vi "Measurement UI.vi"() -> ()   [LabVIEW 2023, in "FPT Framework UI.lvlib"]
uses:
  FPT Framework UI.lvlib
panel:
  in  "Measurement Graph":T1(tab)
  out "General Graph 1":T2(graph)
  out "General Graph 2":T2(graph)
  out "General Graph 3":T2(graph)
  out "General Graph 4":T2(graph)
  out "General Graph 5":T2(graph)
  out "PAE@Pin(s)":string[](array[string])
  out "Gain@Pin(s)":string[](array[string])
  out "Pout@Pin(s)":string[](array[string])
  out "Pout@Pin vs Freq":dbl[][](array[numeric])
  out "PAE vs Pin per Freq":dbl[][](array[numeric])
  out "Gain vs Pin per Freq":dbl[][](array[numeric])
  out "Group B Graph":refnum<vi>[](array[refnum])
  out "Group A Graph":refnum<vi>[](array[refnum])
  in  "Power sequencing file path":string
  out "All Graph Refs":refnum<vi>[](array[refnum])
  out "Pout vs Pin per Freq":dbl[][](array[numeric])
  out "OPxdB vs Freq":dbl[][](array[numeric])
  out "Linear Gain vs Freq":dbl[][](array[numeric])
  out "Frequencies":string[](array[string])
  out "OPxdB(s)":string[](array[string])
  out "Linear Gain(s)":string[](array[string])
  out "Full Data per Frequency":string[][](array[string])
  out "Pin(s)":string[](array[string])
  in  "SMU name":string caption="SMU Name"
  out "Table 2 Header":string[](array[string])
  out "Table 1 Header":string[](array[string])
  out "Gain@Pin vs Freq":dbl[][](array[numeric])
  out "PAE@Pin vs Freq":dbl[][](array[numeric])
  out "MeasTable 1":string[][](table)
  out "MeasTable 2":string[][](table)
  in  "Mode of operation":enum32{"Power Sequence", "Measurement 1"}(ring) caption="Configuration"
  in  "Tab Control":enum32{"Power Sequence", "Measurement 1"}(tab)
  in  "Power sequencing file path_update":path caption="Power Sequencing File Path"
  in  "SMU channel":string caption="SMU Channel"
  in  "SMU name_update":refnum<k15> caption="SMU Name"
  in  "Compression_Target Pin (dBm)":dbl=1.0 caption="Target Pin" format="%#pdBm"
  in  "Compression_Expected DUT Gain (dB)":dbl=17.5 caption="Expected DUT Gain" format="%#pdB"
  in  "Compression_Max Linear Range (dBm)":dbl=-10.0 caption="Max Linear Range" format="%#pdBm"
  in  "Compression_Compression Point (dB)":dbl=1.0 caption="PxdB" format="%#pdB"
  in  "Compression_RFSG Frequency Start (Hz)":dbl=6000000000.0 caption="Frequency Start" step=1000000.0 format="%#pHz"
  in  "Compression_RFSG Power Start (dBm)":dbl=-20.0 caption="Power Start" format="%#pdBm"
  in  "Compression_RFSG Power Step Size (dB)":dbl=1.0 caption="Power Step Size" format="%#pdB"
  in  "Compression_RFSG Power Stop(dBm)":dbl=4.0 caption="Power End" format="%#pdBm"
  in  "Compression_RBW (Hz)":dbl=5000000.0 caption="RBW" format="%#pHz"
  in  "Compression_RFSG Frequency Stop (Hz)":dbl=18000000000.0 caption="Frequency Stop" step=1000000.0 format="%#pHz"
  in  "Compression_RFSG Number of Frequency Step":i32=10 caption="Number of Steps"
  out "Status":string
  # "Frequency Sweep"
  # "Power Sweep"
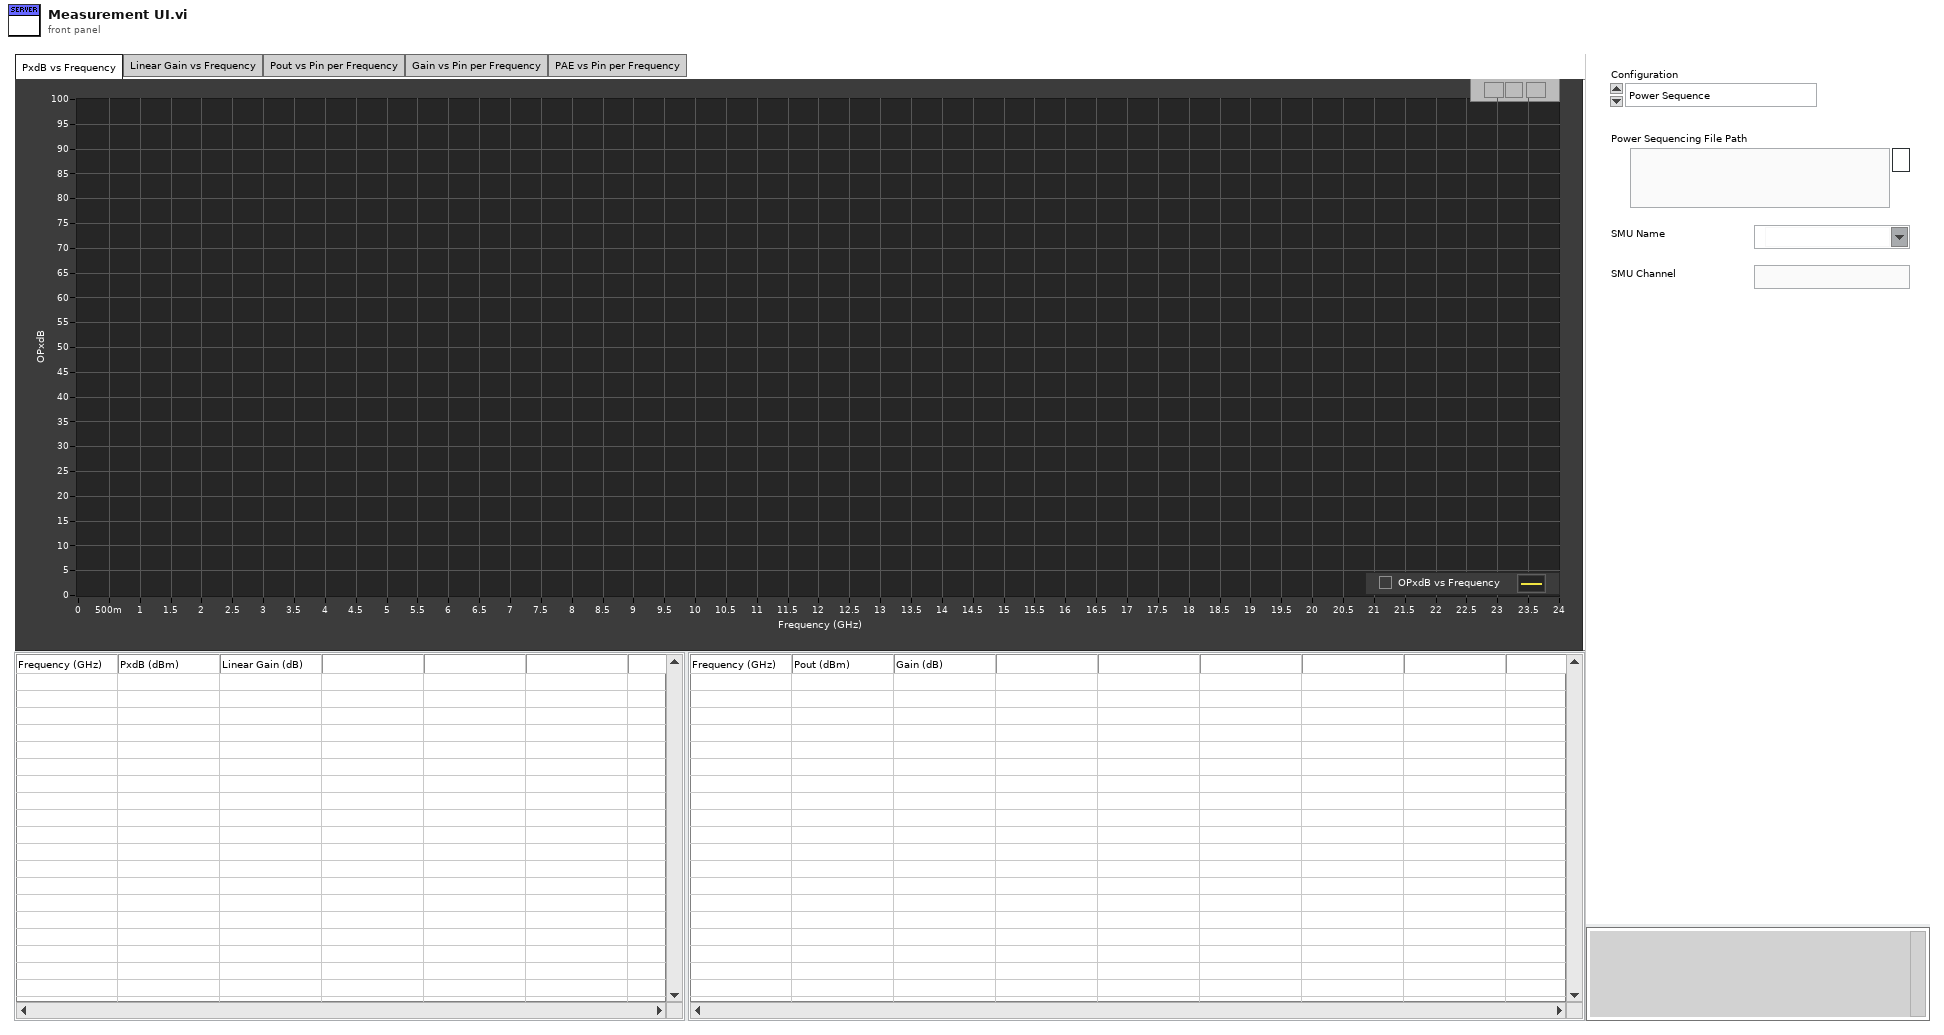
[diagram p1: front panel]
types:
  T1 = enum32{"PxdB vs Frequency", "Linear Gain vs Frequency", "Pout vs Pin per Frequency", "Gain vs Pin per Frequency", "PAE vs Pin per Frequency", "Hidden Controls"}
  T2 = cluster{"Load currents":dbl[], "Efficiency":dbl[]}[]
  T3 = cluster{"Shift":bool, "Ctrl":bool, "Alt":bool, "Cmd":bool, "Opt":bool}
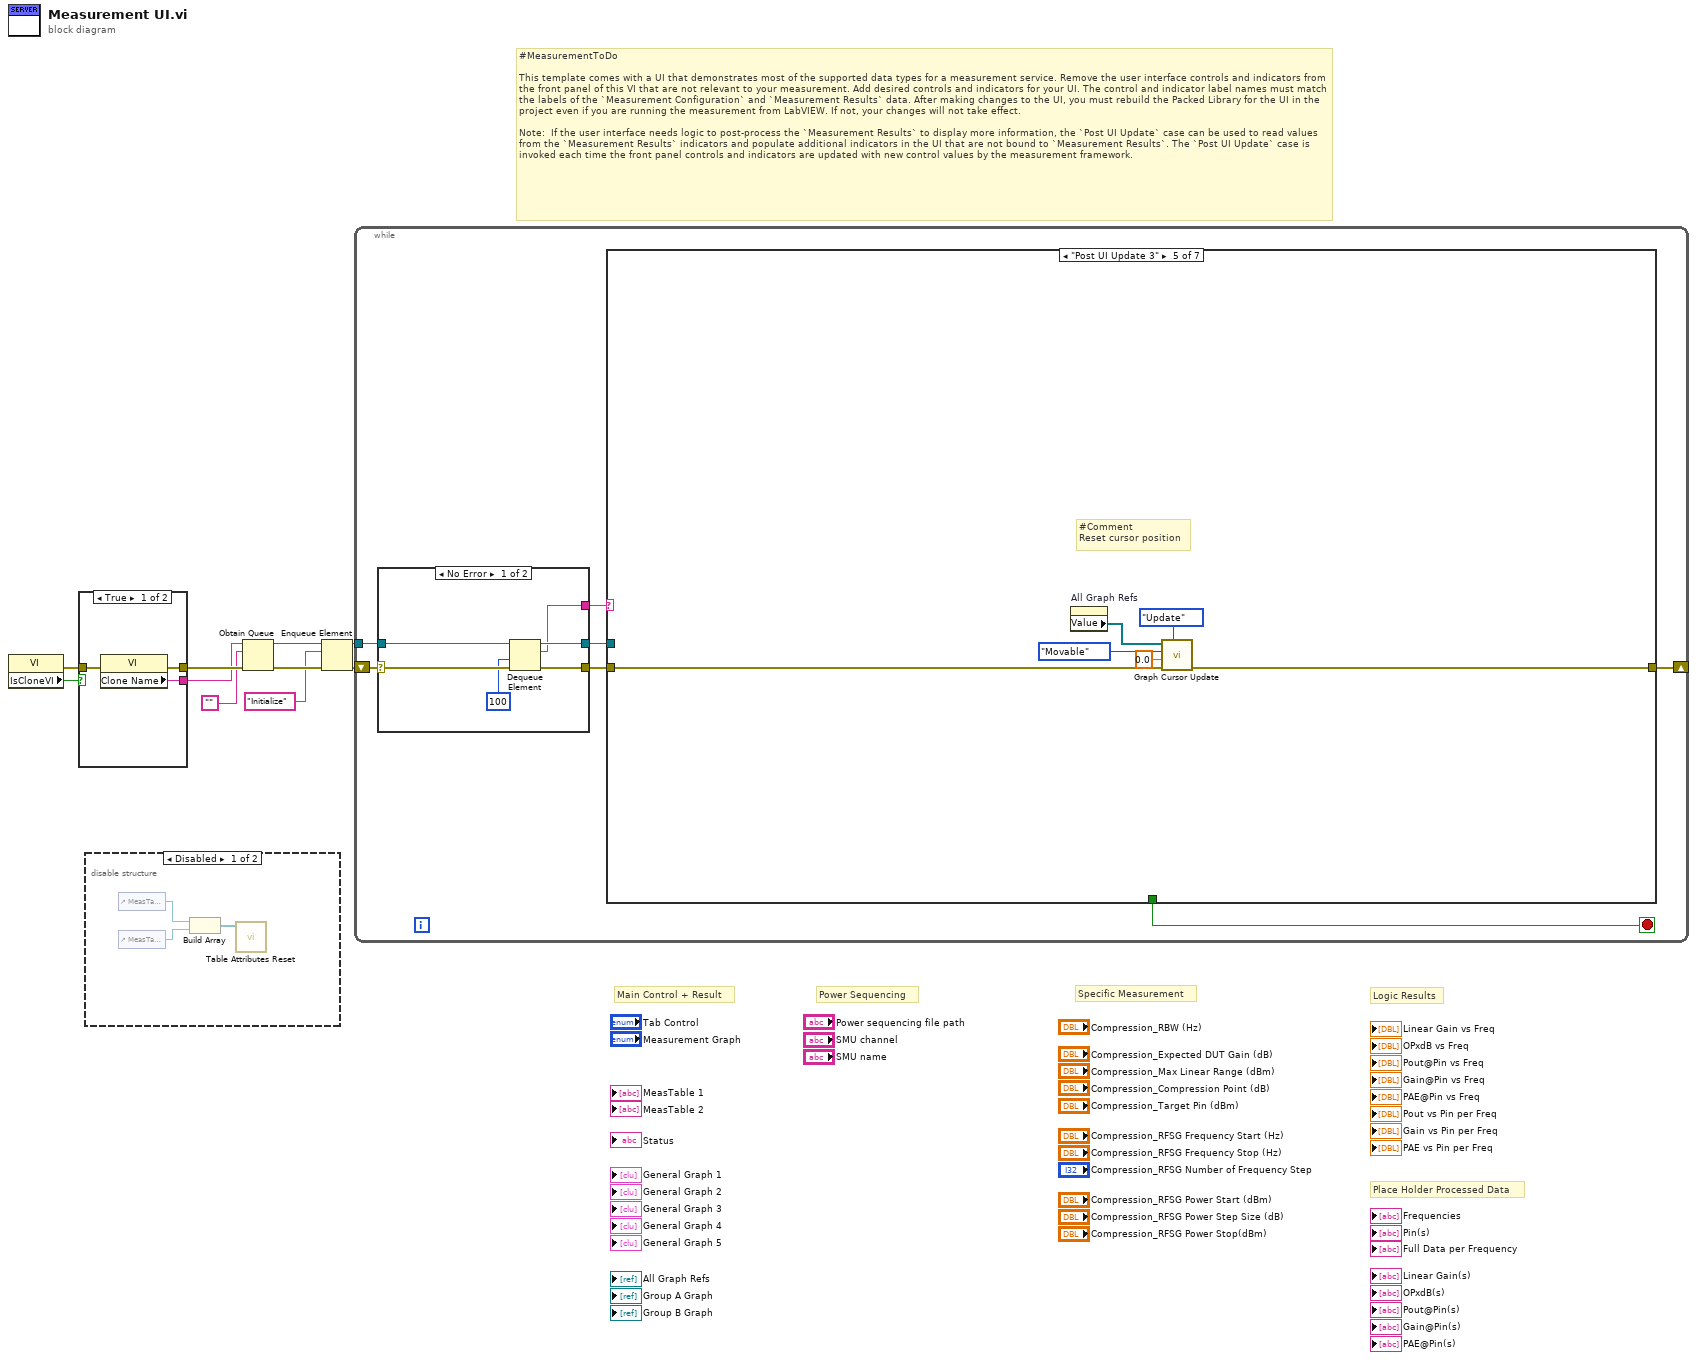
[diagram p0: block diagram]
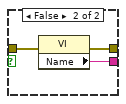
[diagram p3: hidden frame]
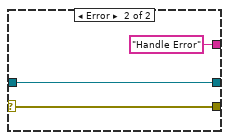
[diagram p4: hidden frame]
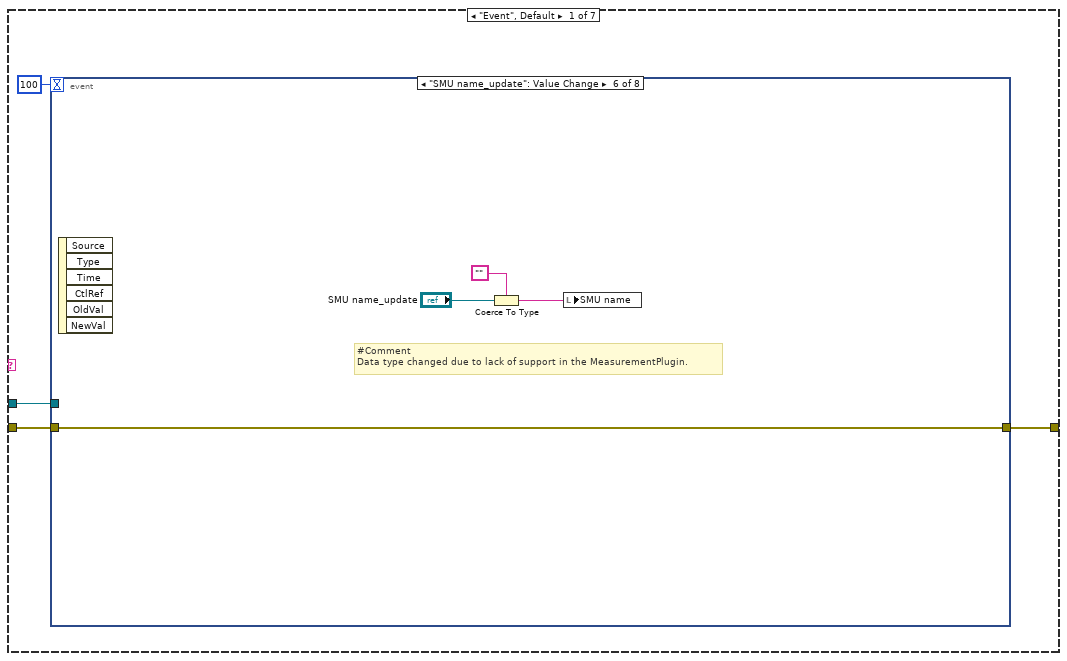
[diagram p5: hidden frame]
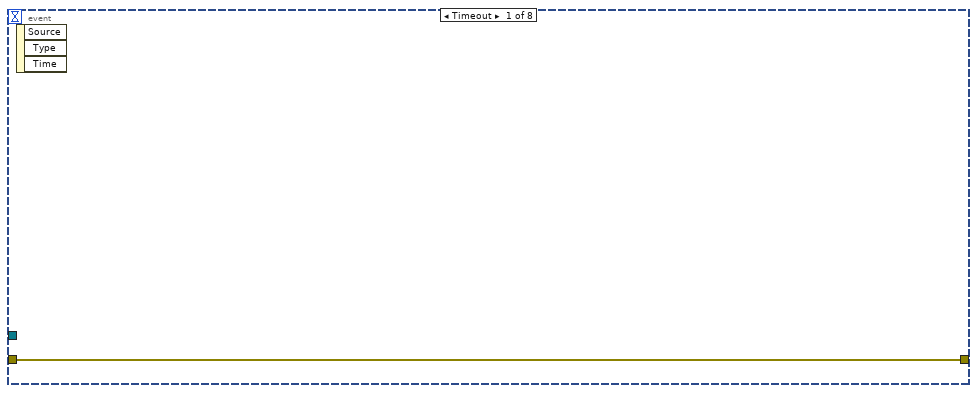
[diagram p6: hidden frame]
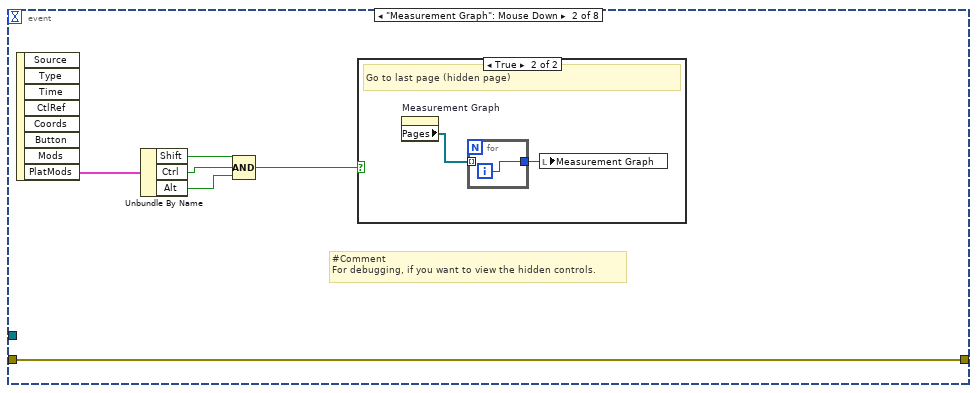
[diagram p7: hidden frame]
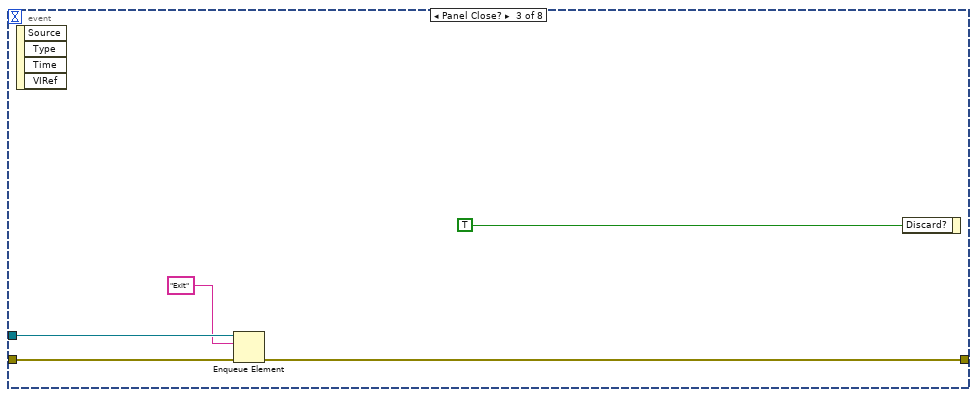
[diagram p9: hidden frame]
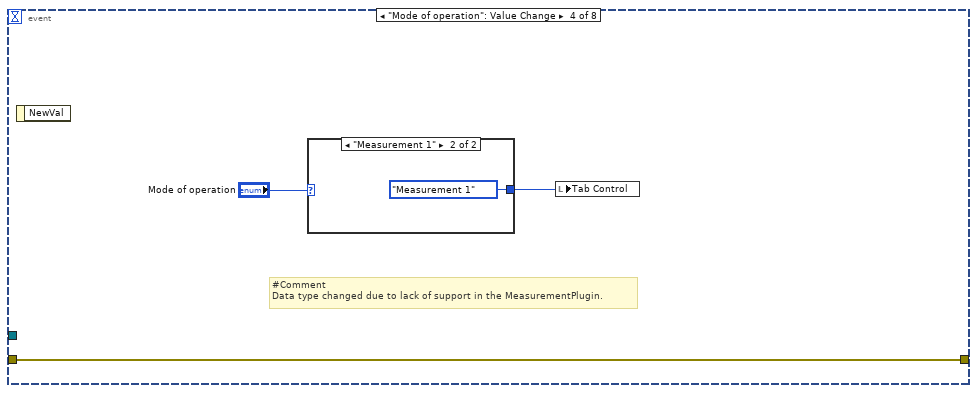
[diagram p10: hidden frame]
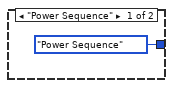
[diagram p11: hidden frame]
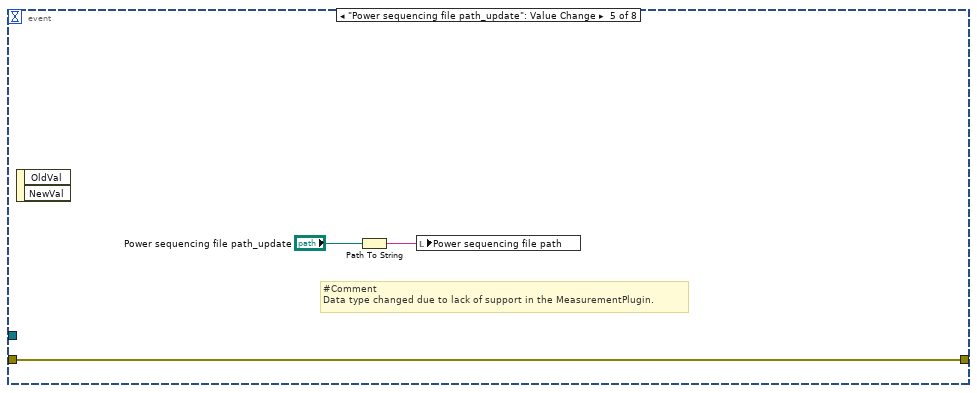
[diagram p12: hidden frame]
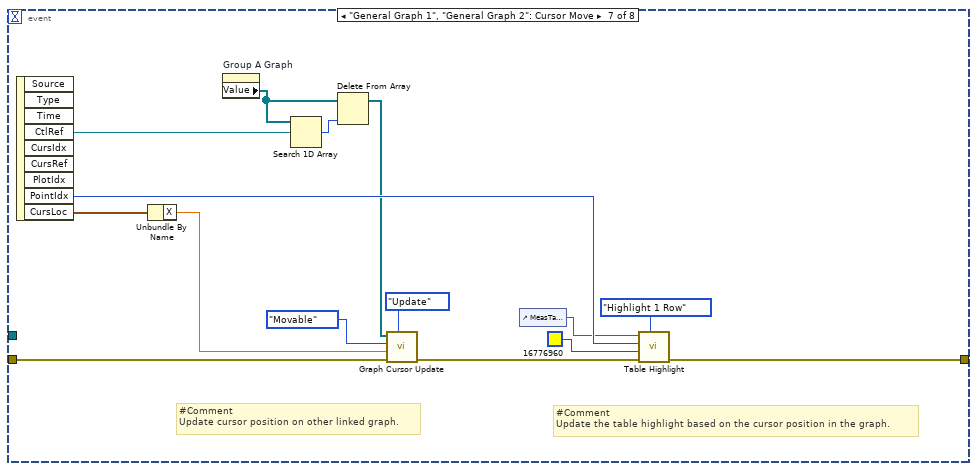
[diagram p13: hidden frame]
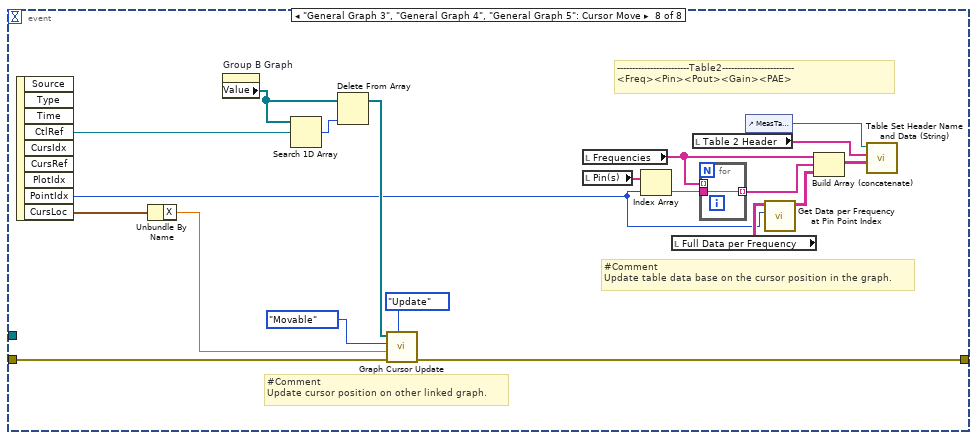
[diagram p14: hidden frame]
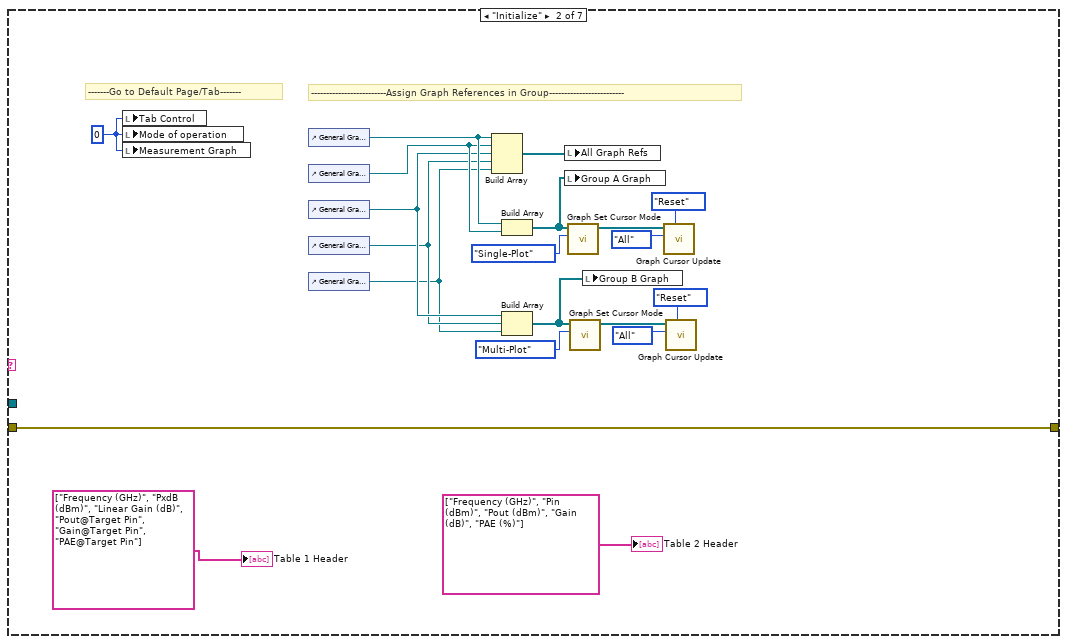
[diagram p15: hidden frame]
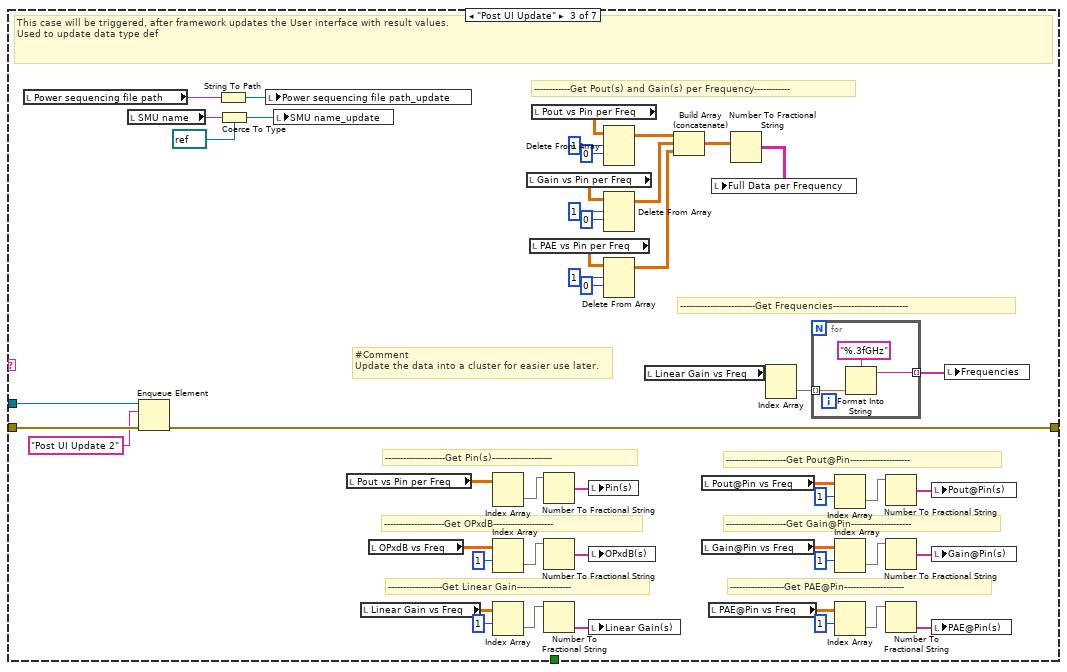
[diagram p16: hidden frame]
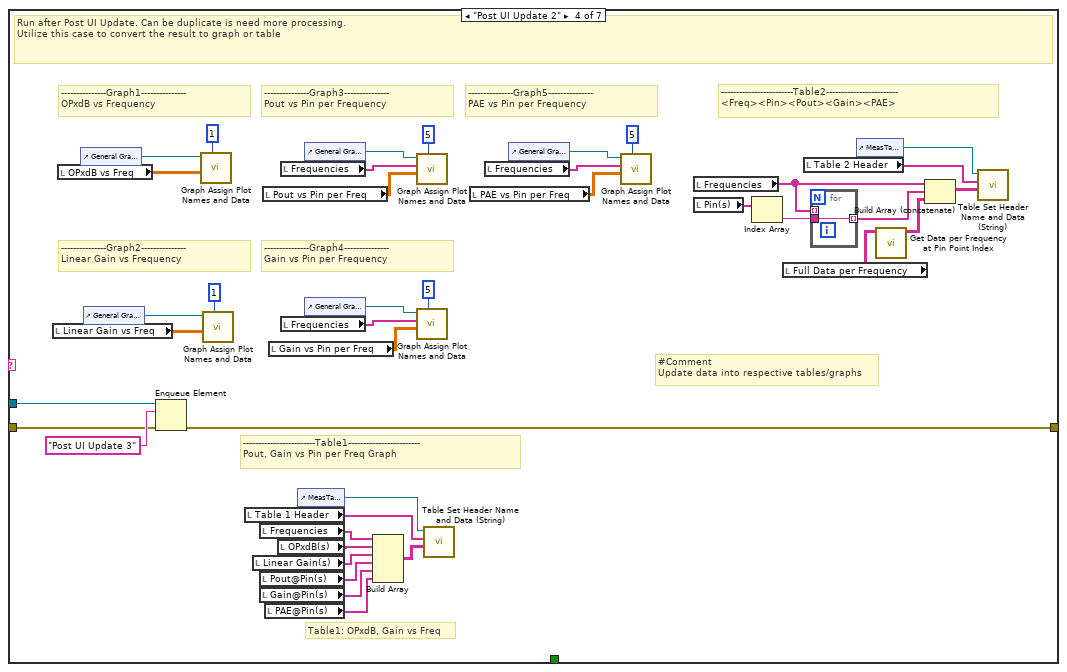
[diagram p17: hidden frame]
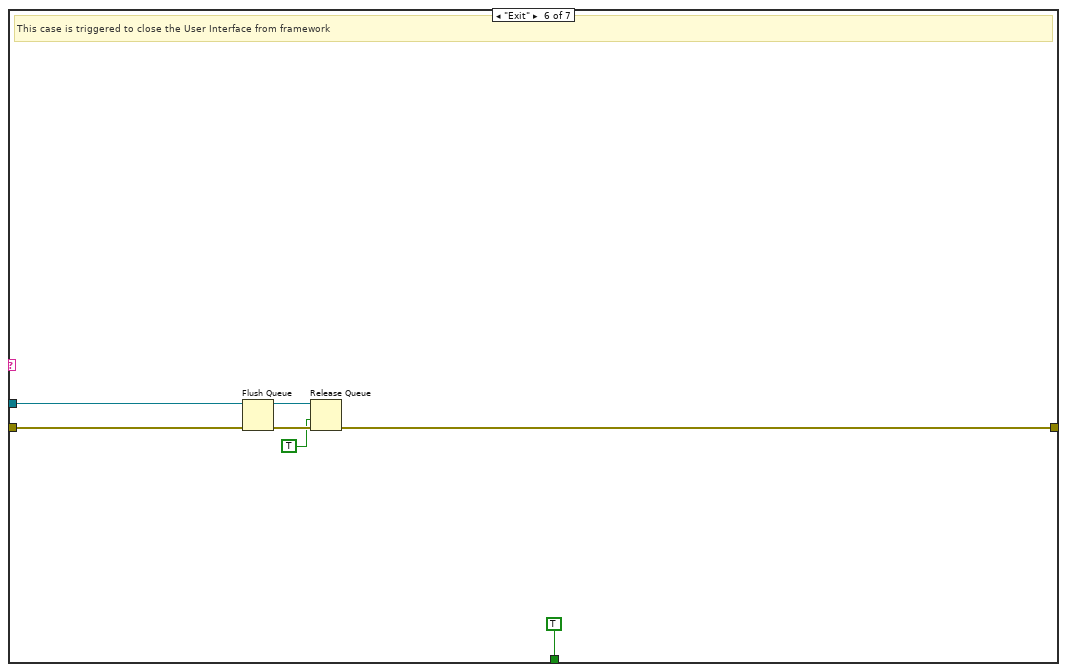
[diagram p18: hidden frame]
diagram:
  # "Logic Results"
  # "Place Holder Processed Data"
  # "Specific Measurement"
  # "Power Sequencing"
  # "Main Control + Result"
  # "#MeasurementToDo  \n\nThis template comes with a UI that demonstrates most of the supported data types for a measurement service. Remove the user interface controls and indicators from the front panel of this VI that are not relevant to your measurement. Add desired controls and indicators for your UI. The control and indicator label names must match the labels of the `Measurement Configuration` and `Measurement Results` data. After making changes to the UI, you must rebuild the Packed Library for the UI in the project even if you are running the measurement from LabVIEW. If not, your changes will not take effect.\n\nNote:  If the user interface needs logic to post-process the `Measurement Results` to display more information, the `Post UI Update` case can be used to read values from the `Measurement Results` indicators and populate additional indicators in the UI that are not bound to `Measurement Results`. The `Post UI Update` case is invoked each time the front panel controls and indicators are updated with new control values by the measurement framework."
  n1 = property class="VI"() -> (error out=w1:errorcluster, "IsCloneVI"=w2:bool)  [unwired: 2 in, 1 out]
  n2 = case shown="True" w2 {
    tunnel: [w13 w16] -> w10
    tunnel: [w12 w15] -> w9
    tunnel: w1 -> [w11 w14]
    frame True {
      n3 = property class="VI"(error in=w11) -> (error out=w13:errorcluster, "Clone Name"=w12:string)  [unwired: 1 in, 1 out]
    }
    frame False {
      n4 = property class="VI"(error in=w14) -> (error out=w16:errorcluster, "Name"=w15:string)  [unwired: 1 in, 1 out]
    }
  }
  n5 = disable-structure shown="Disabled" {
    frame Disabled {
      n6 = control-ref of="MeasTable 2"() -> (w19:refnum<vi>)
      n7 = control-ref of="MeasTable 1"() -> (w18:refnum<vi>)
      n8 = Build Array(w19, w18) -> (w17:refnum<vi>[])
      n9 = call "Table Attributes Reset.vi"("Table Refs"=w17) -> ()  [unwired: 11 in]
    }
    frame Enabled {
    }
  }
  n10 = Obtain Queue(name (unnamed)=w9, element data type="", error in (no error)=w10) -> (queue out=w6:refnum<queue>, error out=w8:errorcluster)  [unwired: 2 in, 1 out]
  n11 = Enqueue Element(queue=w6, element="Initialize", error in (no error)=w8) -> (queue out=w5:refnum<queue>, error out=w7:errorcluster)  [unwired: 1 in, 1 out]
  n12 = while {
    shift-right: [w21] -> _
    shift-left: w7 -> [w26]
    tunnel: w5 -> [w24]
    stop <- w20 stop-if-true
    n13 = case shown="No Error" w26 {
      selector: w26 -> [w32 w35]
      tunnel: [w31 w35] -> w25
      tunnel: w24 -> [w30 w34]
      tunnel: [w29 w34] -> w23
      tunnel: [w28 "Handle Error"] -> w22
      frame No Error {
        n14 = Dequeue Element(queue=w30, timeout in ms (-1)=100, error in (no error)=w32) -> (queue out=w29:refnum<queue>, element=w28:string, error out=w31:errorcluster)  [unwired: 1 out]
      }
      frame Error {
      }
    }
    n15 = case shown="\"Post UI Update 3\"" w22 {
      tunnel: w25 -> [w38 w122 w170 w212 w220 w227 w228]
      tunnel: w23 -> [w36 _ w169 w210 _ w225 _]
      tunnel: [w39 w122 w170 w211 w215 w222 w228] -> w21
      tunnel: [_ _ _ _ _ TRUE _] -> w20
      frame "Event", Default {
        n16 = event shown="[5] \"SMU name_update\": Value Change" {
          selector: _ -> [_ _ _ _ _ _ _ _]
          dyn-events: _ -> [_ _ _ _ _ _ _ _]
          timeout: 100 -> [_ _ _ _ _ _ _ _]
          tunnel: [w40 w41 w52 w56 w60 w66 w79 w100] -> w39
          tunnel: w38 -> [w40 w41 w53 w56 w60 w66 w81 w101]
          tunnel: w36 -> [_ _ w51 _ _ _ _ _]
          event Timeout {
            n17 = event-data() -> ()  [unwired: 1 in, 3 out]
          }
          event "Measurement Graph": Mouse Down {
            # "#Comment\nFor debugging, if you want to view the hidden controls."
            n18 = event-data() -> ("PlatMods"=w46:T3)  [unwired: 1 in, 7 out]
            n19 = Unbundle By Name(w46) -> ("Shift"=w45:bool, "Ctrl"=w44:bool, "Alt"=w43:bool)
            n20 = Compound Arithmetic op=AND(w45, w44, w43) -> (w42:bool)
            n21 = case shown="True" w42 {
              frame False {
              }
              frame True {
                # "Go to last page (hidden page)"
                n22 = property on="Measurement Graph" class="TabCtl (strict)"() -> ("Pages"=w48:refnum<vi>[])  [unwired: 2 in, 2 out]
                n23 = for {
                  tunnel: w48 -> [_] mode=indexing
                  tunnel: [w49] -> w47
                  i -> [w49]
                }
                n24 = local write "Measurement Graph"(w47) -> ()
              }
            }
          }
          event Panel Close? {
            n25 = event-data() -> ()  [unwired: 1 in, 4 out]
            n26 = Enqueue Element(queue=w51, element="Exit", error in (no error)=w53) -> (error out=w52:errorcluster)  [unwired: 1 in, 2 out]
            n27 = event-data("Discard?"=TRUE) -> ()  [unwired: 1 in, 1 out]
          }
          event "Mode of operation": Value Change {
            # "#Comment\nData type changed due to lack of support in the MeasurementPlugin."
            n28 = event-data() -> ()  [unwired: 1 in, 1 out]
            n29 = case shown="\"Measurement 1\"" "Mode of operation" {
              tunnel: [enum32{"Power Sequence", "Measurement 1"}."Power Sequence" ("Tab Control") enum32{"Power Sequence", "Measurement 1"}."Measurement 1" ("Tab Control")] -> w55
              frame "Power Sequence" {
              }
              frame "Measurement 1" {
              }
            }
            n30 = local write "Tab Control"(w55) -> ()
          }
          event "Power sequencing file path_update": Value Change {
            # "#Comment\nData type changed due to lack of support in the MeasurementPlugin."
            n31 = event-data() -> ()  [unwired: 1 in, 2 out]
            n32 = Path To String(path="Power sequencing file path_update") -> (string=w61:string)
            n33 = local write "Power sequencing file path"(w61) -> ()
          }
          event "SMU name_update": Value Change {
            # "#Comment\nData type changed due to lack of support in the MeasurementPlugin."
            n34 = event-data() -> ()  [unwired: 1 in, 6 out]
            n35 = Coerce To Type(0:"SMU name_update", 1:"") -> (2:w63:string)
            n36 = local write "SMU name"(w63) -> ()
          }
          event "General Graph 1", "General Graph 2": Cursor Move {
            # "#Comment\nUpdate cursor position on other linked graph."
            # "#Comment\nUpdate the table highlight based on the cursor position in the graph."
            n37 = event-data() -> ("CtlRef"=w72:refnum<vi>, "PointIdx"=w78:i32, "CursLoc"=w76:cluster{"X":dbl, "Y":dbl})  [unwired: 1 in, 6 out]
            n38 = Unbundle By Name(w76) -> ("X"=w75:dbl)
            n39 = property on="Group A Graph" class="Arr (strict)"() -> ("Value"=w73:refnum<vi>[])  [unwired: 2 in, 2 out]
            n40 = Search 1D Array(1D array=w73, element=w72) -> (index of element=w74:i32)  [unwired: 1 in]
            n41 = Delete From Array(array=w73, index=w74) -> (array with subset deleted=w71:refnum<vi>[])  [unwired: 1 in, 1 out]
            n42 = call "Graph Cursor Update.vi"("Action"=enum16{"Reset", "Update"}."Update", "error in"=w81, "New X position"=w75, "Cursor Type"=enum16{"Movable", "Fixed", "All"}."Movable", "Graph Refs in"=w71) -> ("error out"=w80:errorcluster)  [unwired: 5 in, 1 out]
            n43 = control-ref of="MeasTable 1"() -> (w68:refnum<vi>)
            n44 = call "Table Highlight.vi"("Action"=enum16{"Reset", "Highlight 1 Row"}."Highlight 1 Row", "error in"=w80, "Color Box"=u32 16776960, "Row"=w78, "Table Ref in"=w68) -> ("error out"=w79:errorcluster)  [unwired: 5 in, 1 out]
          }
          event "General Graph 3", "General Graph 4", "General Graph 5": Cursor Move {
            # "#Comment\nUpdate cursor position on other linked graph."
            # "#Comment\nUpdate table data base on the cursor position in the graph."
            # "------------------------Table2------------------------\n<Freq><Pin><Pout><Gain><PAE>"
            n45 = event-data() -> ("CtlRef"=w94:refnum<vi>, "PointIdx"=w84:i32, "CursLoc"=w98:cluster{"X":dbl, "Y":dbl})  [unwired: 1 in, 6 out]
            n46 = Unbundle By Name(w98) -> ("X"=w97:dbl)
            n47 = property on="Group B Graph" class="Arr (strict)"() -> ("Value"=w95:refnum<vi>[])  [unwired: 2 in, 2 out]
            n48 = Search 1D Array(1D array=w95, element=w94) -> (index of element=w96:i32)  [unwired: 1 in]
            n49 = Delete From Array(array=w95, index=w96) -> (array with subset deleted=w93:refnum<vi>[])  [unwired: 1 in, 1 out]
            n50 = call "Graph Cursor Update.vi"("Action"=enum16{"Reset", "Update"}."Update", "error in"=w101, "New X position"=w97, "Cursor Type"=enum16{"Movable", "Fixed", "All"}."Movable", "Graph Refs in"=w93) -> ("error out"=w100:errorcluster)  [unwired: 5 in, 1 out]
            n51 = local read "Frequencies"() -> (w85:string[])
            n52 = local read "Pin(s)"() -> (w88:string[])
            n53 = Index Array(array=w88, index=w84) -> (element=w87:string)
            n54 = local read "Full Data per Frequency"() -> (w89:string[][])
            n55 = local read "Table 2 Header"() -> (w82:string[])
            n56 = for {
              tunnel: [w102] -> w86 mode=indexing
              tunnel: w87 -> [w102]
              tunnel: w85 -> [_] mode=indexing
            }
            n57 = control-ref of="MeasTable 2"() -> (w91:refnum<vi>)
            n58 = call "Get Data per Frequency at Pin Point Index.vi"("Pin Point Index"=w84, "Full Data per Freq"=w89) -> ("Focused Data"=w83:string[][])  [unwired: 9 in]
            n59 = Build Array (concatenate)(w85, w86, w83) -> (w90:string[][])
            n60 = call "Table Set Header Name and Data (String).vi"("Data"=w90, "Header"=w82, "Table Ref"=w91) -> ()  [unwired: 9 in]
          }
        }
      }
      frame "Initialize" {
        w114 = 0
        # "-------Go to Default Page/Tab-------"
        # "-------------------------Assign Graph References in Group-------------------------"
        n61 = local write "Tab Control"(w114) -> ()
        n62 = local write "Mode of operation"(w114) -> ()
        n63 = local write "Measurement Graph"(w114) -> ()
        n64 = control-ref of="General Graph 1"() -> (w117:refnum<vi>)
        n65 = control-ref of="General Graph 2"() -> (w116:refnum<vi>)
        n66 = control-ref of="General Graph 3"() -> (w115:refnum<vi>)
        n67 = control-ref of="General Graph 4"() -> (w106:refnum<vi>)
        n68 = control-ref of="General Graph 5"() -> (w105:refnum<vi>)
        n69 = Build Array(w117, w116, w115, w106, w105) -> (w113:refnum<vi>[])
        n70 = Build Array(w117, w116) -> (w112:refnum<vi>[])
        n71 = Build Array(w115, w106, w105) -> (w107:refnum<vi>[])
        n72 = local write "All Graph Refs"(w113) -> ()
        n73 = local write "Group A Graph"(w112) -> ()
        n74 = call "Graph Set Cursor Mode.vi"("Cursor Mode"=enum32{"Free-Drag", "Single-Plot", "Multi-Plot"}."Single-Plot", "Graph Refs in"=w112) -> ("Graph Refs out"=w118:refnum<vi>[])  [unwired: 8 in, 1 out]
        n75 = call "Graph Set Cursor Mode.vi"("Cursor Mode"=enum32{"Free-Drag", "Single-Plot", "Multi-Plot"}."Multi-Plot", "Graph Refs in"=w107) -> ("Graph Refs out"=w111:refnum<vi>[])  [unwired: 8 in, 1 out]
        n76 = local write "Group B Graph"(w107) -> ()
        n77 = call "Graph Cursor Update.vi"("Action"=enum16{"Reset", "Update"}."Reset", "Cursor Type"=enum16{"Movable", "Fixed", "All"}."All", "Graph Refs in"=w118) -> ()  [unwired: 7 in, 2 out]
        n78 = call "Graph Cursor Update.vi"("Action"=enum16{"Reset", "Update"}."Reset", "Cursor Type"=enum16{"Movable", "Fixed", "All"}."All", "Graph Refs in"=w111) -> ()  [unwired: 7 in, 2 out]
        "Table 2 Header" <- string[] ["Frequency (GHz)", "Pin (dBm)", "Pout (dBm)", "Gain (dB)", "PAE (%)"] ("Header")
        "Table 1 Header" <- string[] ["Frequency (GHz)", "PxdB (dBm)", "Linear Gain (dB)", "Pout@Target Pin", "Gain@Target Pin", "PAE@Target Pin"] ("Header")
      }
      frame "Post UI Update" {
        # "#Comment\nUpdate the data into a cluster for easier use later."
        # "--------------------Get Pout@Pin--------------------"
        # "------------------Get PAE@Pin--------------------"
        # "--------------------Get Gain@Pin--------------------"
        # "------------Get Pout(s) and Gain(s) per Frequency------------"
        # "-------------------------Get Frequencies-------------------------"
        # "------------------Get Linear Gain------------------"
        # "--------------------Get OPxdB--------------------"
        # "--------------------Get Pin(s)--------------------"
        # "This case will be triggered, after framework updates the User interface with result values.\nUsed to update data type def"
        n79 = local read "Power sequencing file path"() -> (w166:string)
        n80 = local read "SMU name"() -> (w141:string)
        n81 = Enqueue Element(queue=w169, element="Post UI Update 2") -> ()  [unwired: 2 in, 3 out]
        n82 = String To Path(string=w166) -> (path=w167:path)
        n83 = Coerce To Type(0:w141, 1:refnum<k15> refnum ("RFSG name_update")) -> (2:w139:refnum<k15>)
        n84 = local write "Power sequencing file path_update"(w167) -> ()
        n85 = local write "SMU name_update"(w139) -> ()
        n86 = local read "Pout vs Pin per Freq"() -> (w162:dbl[][])
        n87 = local read "Linear Gain vs Freq"() -> (w156:dbl[][])
        n88 = local read "OPxdB vs Freq"() -> (w158:dbl[][])
        n89 = Index Array(array=w162) -> (element=w161:dbl[])  [unwired: 2 in]
        n90 = Index Array(array=w158, index (row)=1) -> (element=w155:dbl[])  [unwired: 1 in]
        n91 = Index Array(array=w156, index (row)=1) -> (element=w153:dbl[])  [unwired: 1 in]
        n92 = local read "Gain vs Pin per Freq"() -> (w147:dbl[][])
        n93 = local read "PAE vs Pin per Freq"() -> (w136:dbl[][])
        n94 = local read "Pout vs Pin per Freq"() -> (w146:dbl[][])
        n95 = Number To Fractional String(number=w161) -> (F-format string=w160:string[])  [unwired: 3 in]
        n96 = Number To Fractional String(number=w155) -> (F-format string=w154:string[])  [unwired: 3 in]
        n97 = Number To Fractional String(number=w153) -> (F-format string=w152:string[])  [unwired: 3 in]
        n98 = local write "Pin(s)"(w160) -> ()
        n99 = local write "OPxdB(s)"(w154) -> ()
        n100 = local write "Linear Gain(s)"(w152) -> ()
        n101 = Delete From Array(array=w146, length=1, index (row)=0) -> (array with subset deleted=w148:dbl[][])  [unwired: 1 in, 1 out]
        n102 = Delete From Array(array=w147, length=1, index (row)=0) -> (array with subset deleted=w149:dbl[][])  [unwired: 1 in, 1 out]
        n103 = Delete From Array(array=w136, length=1, index (row)=0) -> (array with subset deleted=w135:dbl[][])  [unwired: 1 in, 1 out]
        n104 = local read "Linear Gain vs Freq"() -> (w165:dbl[][])
        n105 = Build Array (concatenate)(w148, w149, w135) -> (w150:dbl[][])
        n106 = local read "Pout@Pin vs Freq"() -> (w125:dbl[][])
        n107 = local read "Gain@Pin vs Freq"() -> (w128:dbl[][])
        n108 = local read "PAE@Pin vs Freq"() -> (w130:dbl[][])
        n109 = Number To Fractional String(number=w150) -> (F-format string=w151:string[][])  [unwired: 3 in]
        n110 = local write "Full Data per Frequency"(w151) -> ()
        n111 = Index Array(array=w165) -> (element=w164:dbl[])  [unwired: 2 in]
        n112 = for {
          tunnel: w164 -> [w173] mode=indexing
          tunnel: [w171] -> w163 mode=indexing
          # "Get Plot Names"
          n113 = Format Into String(format string="%.3fGHz", w173) -> (resulting string=w171:string)  [unwired: 2 in, 1 out]
        }
        n114 = Index Array(array=w125, index (row)=1) -> (element=w124:dbl[])  [unwired: 1 in]
        n115 = Index Array(array=w128, index (row)=1) -> (element=w131:dbl[])  [unwired: 1 in]
        n116 = Index Array(array=w130, index (row)=1) -> (element=w133:dbl[])  [unwired: 1 in]
        n117 = Number To Fractional String(number=w124) -> (F-format string=w123:string[])  [unwired: 3 in]
        n118 = Number To Fractional String(number=w131) -> (F-format string=w132:string[])  [unwired: 3 in]
        n119 = Number To Fractional String(number=w133) -> (F-format string=w134:string[])  [unwired: 3 in]
        n120 = local write "Pout@Pin(s)"(w123) -> ()
        n121 = local write "Gain@Pin(s)"(w132) -> ()
        n122 = local write "PAE@Pin(s)"(w134) -> ()
        n123 = local write "Frequencies"(w163) -> ()
      }
      frame "Post UI Update 2" {
        # "#Comment\nUpdate data into respective tables/graphs"
        # "---------------Graph5---------------\nPAE vs Pin per Frequency"
        # "---------------Graph2---------------\nLinear Gain vs Frequency"
        # "---------------Graph1---------------\nOPxdB vs Frequency"
        # "---------------Graph4---------------\nGain vs Pin per Frequency"
        # "---------------Graph3---------------\nPout vs Pin per Frequency"
        # "------------------------Table1------------------------\nPout, Gain vs Pin per Freq Graph"
        # "------------------------Table2------------------------\n<Freq><Pin><Pout><Gain><PAE>"
        # "Table1: OPxdB, Gain vs Freq"
        # "Run after Post UI Update. Can be duplicate is need more processing.\nUtilize this case to convert the result to graph or table"
        n124 = local read "Linear Gain vs Freq"() -> (w198:dbl[][])
        n125 = local read "OPxdB vs Freq"() -> (w200:dbl[][])
        n126 = control-ref of="General Graph 1"() -> (w201:refnum<vi>)
        n127 = control-ref of="General Graph 2"() -> (w199:refnum<vi>)
        n128 = Enqueue Element(queue=w210, element="Post UI Update 3", error in (no error)=w212) -> (error out=w211:errorcluster)  [unwired: 1 in, 2 out]
        n129 = call "Graph Assign Plot Names and Data.vi"("Legend Number of Rows"=1, "X Ys Data"=w200, "Graph Ref in"=w201) -> ()  [unwired: 6 in, 3 out]
        n130 = call "Graph Assign Plot Names and Data.vi"("Legend Number of Rows"=1, "X Ys Data"=w198, "Graph Ref in"=w199) -> ()  [unwired: 6 in, 3 out]
        n131 = local read "Table 1 Header"() -> (w177:string[])
        n132 = local read "Linear Gain(s)"() -> (w192:string[])
        n133 = local read "Frequencies"() -> (w194:string[])
        n134 = local read "Pout@Pin(s)"() -> (w176:string[])
        n135 = local read "Gain@Pin(s)"() -> (w175:string[])
        n136 = local read "Pout vs Pin per Freq"() -> (w191:dbl[][])
        n137 = local read "PAE@Pin(s)"() -> (w174:string[])
        n138 = local read "Gain vs Pin per Freq"() -> (w205:dbl[][])
        n139 = local read "OPxdB(s)"() -> (w193:string[])
        n140 = local read "Frequencies"() -> (w185:string[])
        n141 = local read "Frequencies"() -> (w184:string[])
        n142 = control-ref of="MeasTable 1"() -> (w202:refnum<vi>)
        n143 = control-ref of="General Graph 3"() -> (w209:refnum<vi>)
        n144 = control-ref of="General Graph 4"() -> (w206:refnum<vi>)
        n145 = Build Array(w194, w193, w192, w176, w175, w174) -> (w195:string[][])
        n146 = call "Graph Assign Plot Names and Data.vi"("Legend Number of Rows"=5, "X Ys Data"=w191, "Plot Names"=w185, "Graph Ref in"=w209) -> ()  [unwired: 5 in, 3 out]
        n147 = call "Graph Assign Plot Names and Data.vi"("Legend Number of Rows"=5, "X Ys Data"=w205, "Plot Names"=w184, "Graph Ref in"=w206) -> ()  [unwired: 5 in, 3 out]
        n148 = call "Table Set Header Name and Data (String).vi"("Data"=w195, "Header"=w177, "Table Ref"=w202) -> ()  [unwired: 9 in]
        n149 = local read "PAE vs Pin per Freq"() -> (w182:dbl[][])
        n150 = local read "Frequencies"() -> (w183:string[])
        n151 = control-ref of="General Graph 5"() -> (w180:refnum<vi>)
        n152 = call "Graph Assign Plot Names and Data.vi"("Legend Number of Rows"=5, "X Ys Data"=w182, "Plot Names"=w183, "Graph Ref in"=w180) -> ()  [unwired: 5 in, 3 out]
        n153 = local read "Frequencies"() -> (w186:string[])
        n154 = local read "Pin(s)"() -> (w189:string[])
        n155 = Index Array(array=w189) -> (element=w188:string)  [unwired: 1 in]
        n156 = local read "Full Data per Frequency"() -> (w190:string[][])
        n157 = local read "Table 2 Header"() -> (w178:string[])
        n158 = for {
          tunnel: [w214] -> w187 mode=indexing
          tunnel: w188 -> [w214]
          tunnel: w186 -> [_] mode=indexing
        }
        n159 = control-ref of="MeasTable 2"() -> (w204:refnum<vi>)
        n160 = call "Get Data per Frequency at Pin Point Index.vi"("Full Data per Freq"=w190) -> ("Focused Data"=w179:string[][])  [unwired: 10 in]
        n161 = Build Array (concatenate)(w186, w187, w179) -> (w203:string[][])
        n162 = call "Table Set Header Name and Data (String).vi"("Data"=w203, "Header"=w178, "Table Ref"=w204) -> ()  [unwired: 9 in]
      }
      frame "Post UI Update 3" {
        # "#Comment\nReset cursor position"
        n163 = property on="All Graph Refs" class="Arr (strict)"() -> ("Value"=w219:refnum<vi>[])  [unwired: 2 in, 2 out]
        n164 = call "Graph Cursor Update.vi"("Action"=enum16{"Reset", "Update"}."Update", "error in"=w220, "New X position"=0.0, "Cursor Type"=enum16{"Movable", "Fixed", "All"}."Movable", "Graph Refs in"=w219) -> ("error out"=w215:errorcluster)  [unwired: 5 in, 1 out]
      }
      frame "Exit" {
        # "This case is triggered to close the User Interface from framework"
        n165 = Flush Queue(queue=w225, error in (no error)=w227) -> (queue out=w224:refnum<queue>, error out=w223:errorcluster)  [unwired: 1 out]
        n166 = Release Queue(queue=w224, force destroy? (F)=TRUE, error in (no error)=w223) -> (error out=w222:errorcluster)  [unwired: 2 out]
      }
      frame "Handle Error" {
      }
    }
  }
